vi "2_3 (SubVI).vi"(1 "Таблиця 1 - Вхідні дані":string[][](table), 2 "Сортувати стовпчик":i32) -> (0 "Таблиця 2 - Результат":string[][](table))   [LabVIEW 2012]
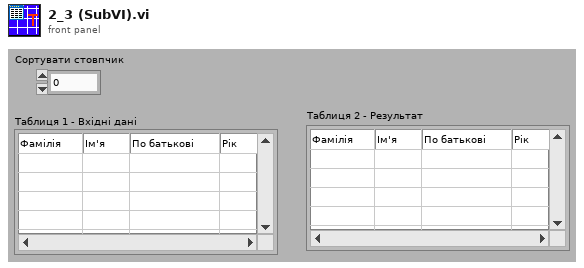
[diagram p1: front panel]
types:
  T1 = cluster{"[0]":string, "[1]":string, "[2]":string, "[3]":string, "[4]":string, "[5]":string, "[6]":string, "[7]":string, "[8]":string}
  T2 = cluster{"[0]":string, "[1]":string, "[2]":string, "[3]":string, "[4]":string, "[5]":string, "[6]":string, "[7]":string, "[8]":string}[]
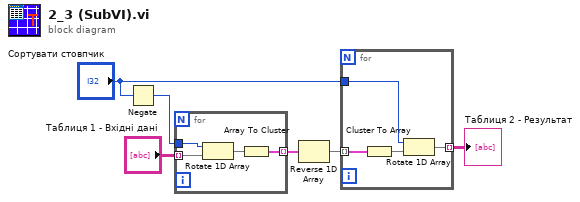
[diagram p0: block diagram]
diagram:
  n1 = Negate(x="Сортувати стовпчик") -> (-x=w4:i32)
  n2 = for {
    tunnel: [w10] -> w2 mode=indexing
    tunnel: "Таблиця 1 - Вхідні дані" -> [w8] mode=indexing
    tunnel: w4 -> [w7]
    n3 = Rotate 1D Array(1:w8, 2:w7) -> (0:w9:string[])
    n4 = Array To Cluster(array=w9) -> (cluster=w10:T1)
  }
  n5 = Reverse 1D Array(array=w2) -> (reversed array=w1:T2)
  n6 = for {
    tunnel: w1 -> [w13] mode=indexing
    tunnel: "Сортувати стовпчик" -> [w12]
    tunnel: [w11] -> w6 mode=indexing
    n7 = Cluster To Array(cluster=w13) -> (array=w14:string[])
    n8 = Rotate 1D Array(1:w14, 2:w12) -> (0:w11:string[])
  }
  "Таблиця 2 - Результат" <- w6
